vi "quiz 3.2.vi"() -> ()   [LabVIEW 2017]
panel:
  out "x .and. y?":bool
  out "output string":string
  out "array":string[][](array[string])
  out "Tab Control":T1(tab)
  in  "Ingresar":bool
  in  "usuario":string
  in  "Contraseña":string
  in  "eliminar":bool
  in  "agregar":bool
  in  "añadir":bool
  in  "contraseña":string
  in  "usuario":string
  in  "Quitar":bool
  in  "usuario a eliminar":string
  out "Seccion Inicada por:":string
  # "¿QUE DESEA REALIZAR?"
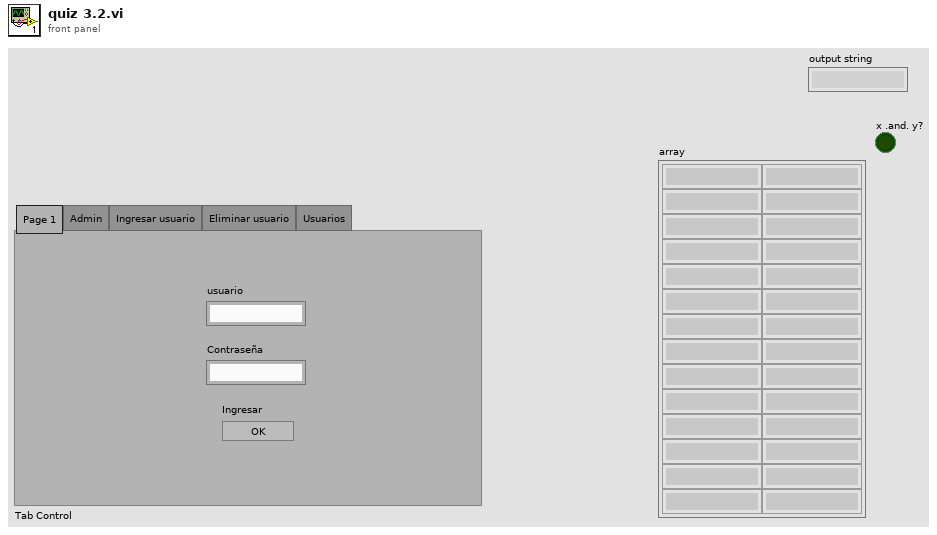
[diagram p1: front panel]
types:
  T1 = enum32{"Page 1", "Admin", "Ingresar usuario", "Eliminar usuario", "Usuarios"}
  T2 = enum16{"open", "replace", "create", "open or create", "replace or create", "replace or create with confirmation"}
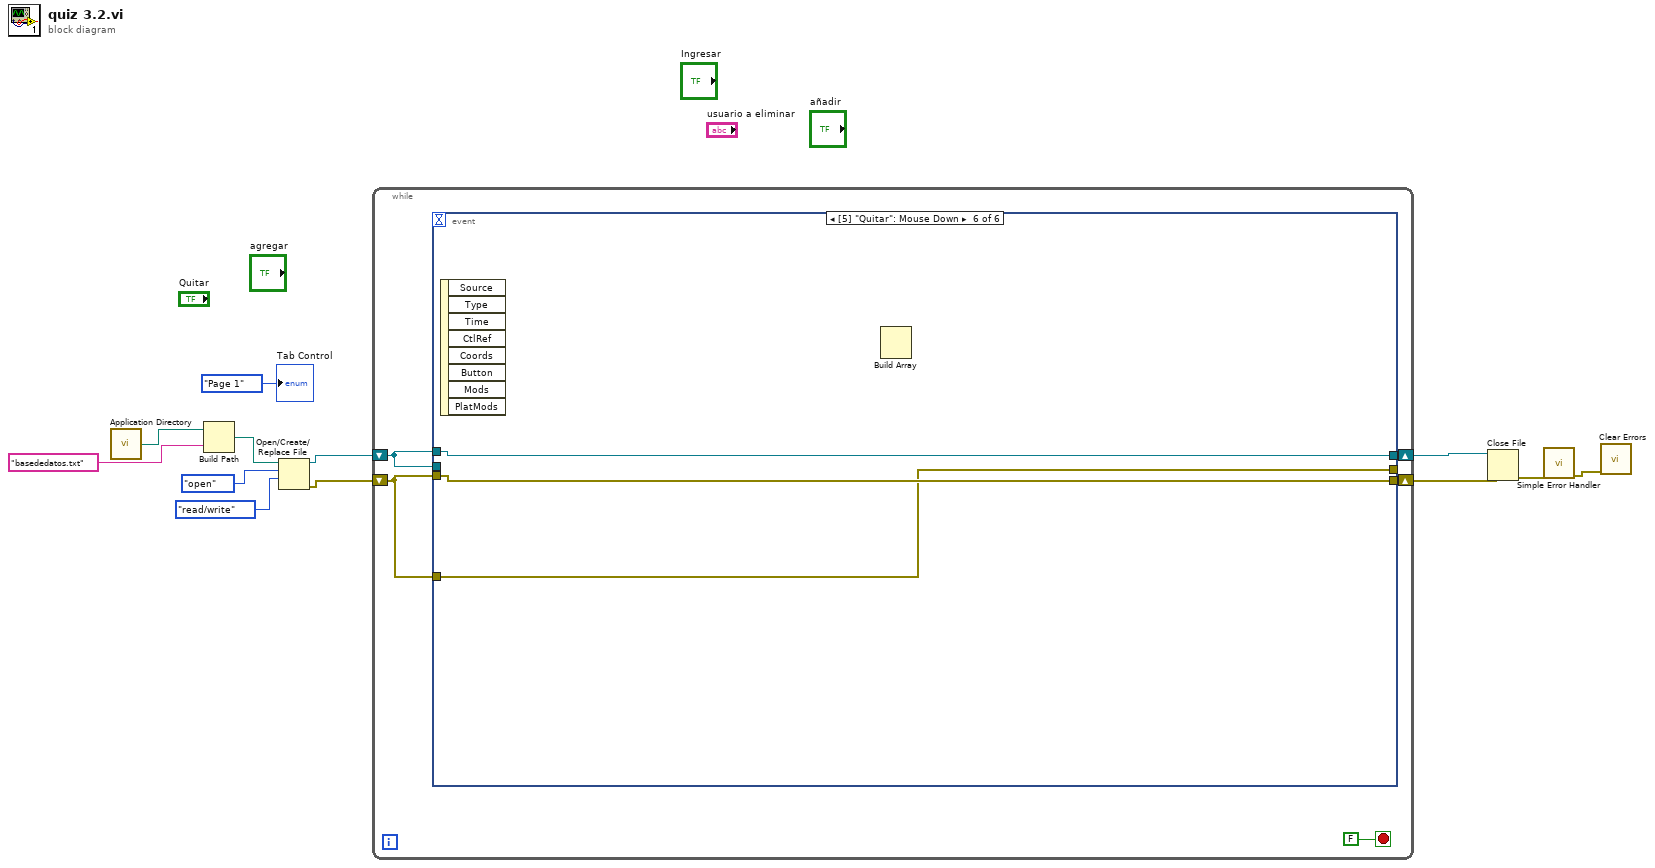
[diagram p0: block diagram]
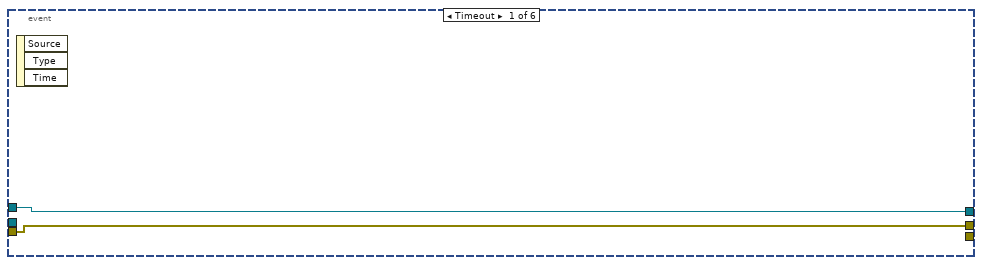
[diagram p2: hidden frame]
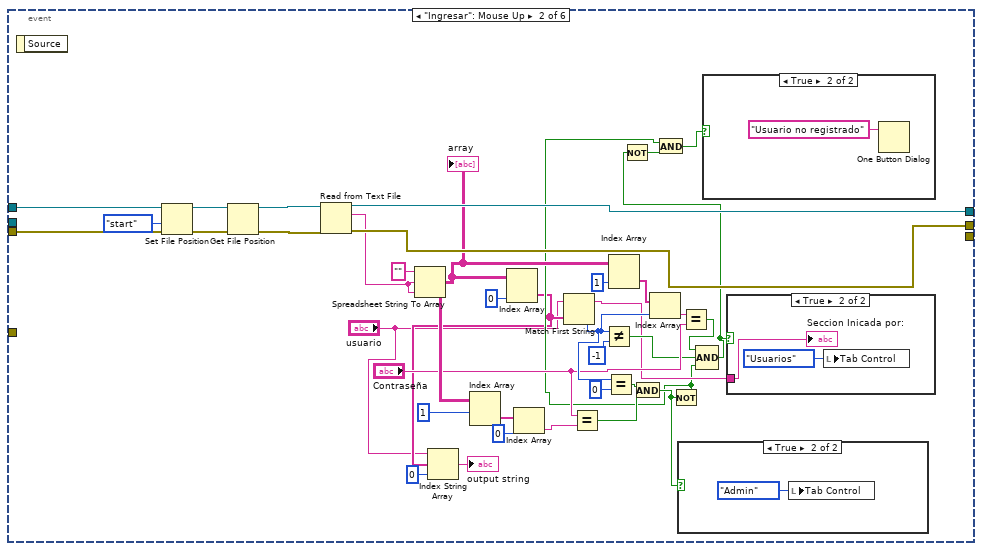
[diagram p3: hidden frame]
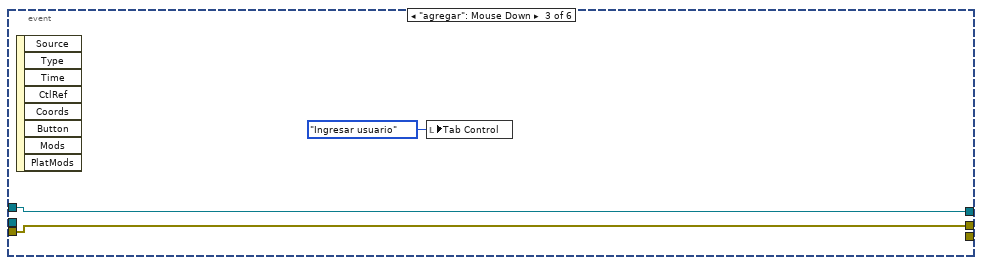
[diagram p7: hidden frame]
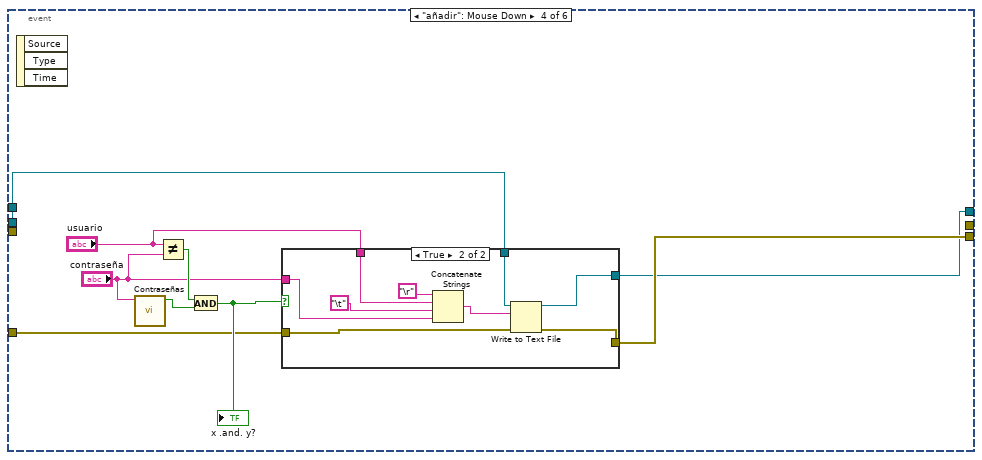
[diagram p8: hidden frame]
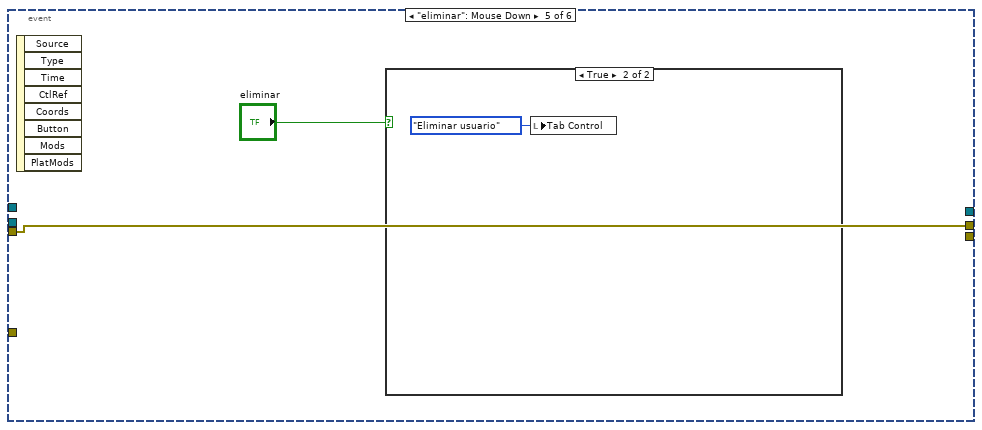
[diagram p10: hidden frame]
diagram:
  n1 = call <vilib>:"Application Directory.vi"() -> ("Application Directory"=w9:path)
  n2 = Build Path(base path=w9, name or relative path="basededatos.txt") -> (appended path=w6:path)
  n3 = Open/Create/Replace File(file path (use dialog)=w6, operation (0:open)=T2."open", access (0:read/write)=enum16{"read/write", "read-only", "write-only"}."read/write") -> (refnum out=w7:refnum<file>, error out=w4:errorcluster)  [unwired: 3 in, 1 out]
  n4 = while {
    shift-right: [w13] -> w10
    shift-left: w7 -> [w15]
    shift-right: [w14] -> w5
    shift-left: w4 -> [w16]
    stop <- FALSE stop-if-true
    n5 = event shown="[5] \"Quitar\": Mouse Down" {
      selector: _ -> [_ _ _ _ _ _]
      dyn-events: _ -> [_ _ _ _ _ _]
      timeout: _ -> [_ _ _ _ _ _]
      tunnel: w15 -> [w19 w53 w64 _ _ w88]
      tunnel: [w19 w52 w64 w65 _ w88] -> w13
      tunnel: [w18 w51 w63 _ w85 w89] -> _
      tunnel: w16 -> [w18 w47 w63 _ w85 w90]
      tunnel: w16 -> [_ _ _ w70 _ w89]
      tunnel: w15 -> [_ _ _ w69 _ _]
      tunnel: [_ _ _ w68 _ w90] -> w14
      event Timeout {
        n6 = event-data() -> ()  [unwired: 1 in, 3 out]
      }
      event "Ingresar": Mouse Up {
        n7 = event-data() -> ()  [unwired: 1 in, 1 out]
        n8 = Set File Position(refnum=w53, from (0:start)=enum16{"start", "end", "current"}."start", error in=w47) -> (refnum out=w57:refnum<file>, error out=w55:errorcluster)  [unwired: 1 in]
        n9 = Get File Position(4:w55, 7:w57) -> (0:w54:errorcluster, 3:w56:refnum<file>)  [unwired: 1 out]
        n10 = Read from Text File(file (use dialog)=w56, error in=w54) -> (refnum out=w52:refnum<file>, text=w49:string, error out=w51:errorcluster)  [unwired: 2 in, 1 out]
        n11 = Spreadsheet String To Array(format string="", spreadsheet string=w49, array type (2D Dbl)=w49) -> (array=w36:string[][])  [unwired: 1 in]
        "array" <- w36
        n12 = Index Array(array=w36, index (col)=1 ("disabled index (col)")) -> (element=w41:string[])  [unwired: 1 in]
        n13 = Index Array(array=w36, index (col)=0 ("disabled index (col)")) -> (element=w23:string[])  [unwired: 1 in]
        n14 = Index String Array(1:0 ("index"), 2:w23, 3:"usuario") -> (0:→"output string":string)
        n15 = Index Array(array=w41, index=0) -> (element=w39:string)
        n16 = Match First String(2:w23, 3:"usuario") -> (0:w33:i32, 1:w25:string)
        n17 = Equal?(x="Contraseña", y=w39) -> (x = y?=w38:bool)
        n18 = Not Equal?(x=w33, y=-1) -> (x != y?=w29:bool)
        n19 = Equal?(x=w33, y=0) -> (x = y?=w43:bool)
        n20 = Index Array(array=w36, index (col)=1 ("disabled index (col)")) -> (element=w34:string[])  [unwired: 1 in]
        n21 = And(x=w43, y=w38) -> (x .and. y?=w37:bool)
        n22 = Index Array(array=w34, index=w33) -> (element=w32:string)
        n23 = Not(x=w37) -> (.not. x?=w24:bool)
        n24 = case shown="True" w37 {
          frame False {
          }
          frame True {
            n25 = local write "Tab Control"(T1."Admin" ("Tab Control")) -> ()
          }
        }
        n26 = Equal?(x=w32, y="Contraseña") -> (x = y?=w30:bool)
        n27 = Compound Arithmetic op=AND(w30, w29, w24) -> (w27:bool)
        n28 = Not(x=w27) -> (.not. x?=w28:bool)
        n29 = And(x=w24, y=w28) -> (x .and. y?=w26:bool)
        n30 = case shown="True" w26 {
          frame False {
          }
          frame True {
            n31 = One Button Dialog(message="Usuario no registrado") -> ()  [unwired: 1 in, 1 out]
          }
        }
        n32 = case shown="True" w27 {
          tunnel: w25 -> [_ w59]
          frame False {
          }
          frame True {
            n33 = local write "Tab Control"(T1."Usuarios" ("Tab Control")) -> ()
            "Seccion Inicada por:" <- w59
          }
        }
      }
      event "agregar": Mouse Down {
        n34 = event-data() -> ()  [unwired: 1 in, 8 out]
        n35 = local write "Tab Control"(T1."Ingresar usuario" ("Tab Control")) -> ()
      }
      event "añadir": Mouse Down {
        n36 = event-data() -> ()  [unwired: 1 in, 3 out]
        n37 = call "Contraseñas.vi"("String"="contraseña") -> ("Contraseña Correcta?"=w73:bool)  [unwired: 10 in]
        n38 = Not Equal?(x="usuario", y="contraseña") -> (x != y?=w72:bool)
        n39 = And(x=w72, y=w73) -> (x .and. y?=w71:bool)
        "x .and. y?" <- w71
        n40 = case shown="True" w71 {
          tunnel: w70 -> [w75 w84]
          tunnel: w69 -> [w74 w83]
          tunnel: [w75 w82] -> w68
          tunnel: [w74 w81] -> w65
          tunnel: "usuario" -> [_ w80]
          tunnel: "contraseña" -> [_ w79]
          frame False {
          }
          frame True {
            n41 = Concatenate Strings("\r", w80, "\t", w79) -> (w78:string)
            n42 = Write to Text File(file (use dialog)=w83, text=w78, error in=w84) -> (refnum out=w81:refnum<file>, error out=w82:errorcluster)  [unwired: 1 in, 1 out]
          }
        }
      }
      event "eliminar": Mouse Down {
        n43 = event-data() -> ()  [unwired: 1 in, 8 out]
        n44 = case shown="True" "eliminar" {
          frame False {
          }
          frame True {
            n45 = local write "Tab Control"(T1."Eliminar usuario" ("Tab Control")) -> ()
          }
        }
      }
      event "Quitar": Mouse Down {
        n46 = event-data() -> ()  [unwired: 1 in, 8 out]
        n47 = Build Array() -> ()  [unwired: 4 in, 1 out]
      }
    }
  }
  n48 = Close File(refnum=w10, error in=w5) -> (error out=w3:errorcluster)  [unwired: 1 out]
  n49 = call <vilib>:"Simple Error Handler.vi"("error in (no error)"=w3) -> ("error out"=w2:errorcluster)  [unwired: 4 in, 4 out]
  n50 = call <vilib>:"Clear Errors.vi"("error in (no error)"=w2) -> ()  [unwired: 5 in, 2 out]
  "Tab Control" <- T1."Page 1" ("Tab Control")
